vi "Global Motor Axis.vi"() -> ()   [LabVIEW 2014]
panel:
  in  "Motor Axis Y":i32
  in  "Motor Axis X":i32
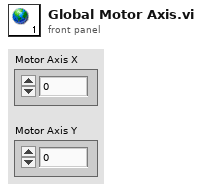
[diagram p1: front panel]
diagram:
